vi "RTS Door Operation Routine.vi"(4 "Relay Number":u8=1 min=1 max=3 step=1, 6 "Station #":u8=1 min=1 max=8 step=1, 8 "Error In":errorcluster, 11 "Door Opening Controller Input":T1 {"Chamber 1-1"."Start Time" format="%<%X\n%x>T"; "Chamber 1-1"."End Time" format="%<%X\n%x>T"; "Time Count (s)" format="%.2f"}) -> (0 "Error Out":errorcluster, 3 "Door Opening Controller Output":T1 {"Chamber 1-1"."Start Time" format="%<%X\n%x>T"; "Chamber 1-1"."End Time" format="%<%X\n%x>T"; "Time Count (s)" format="%.2f"})   [LabVIEW 2016]
uses:
  Type Definitions/RTS Door Opener Indicator.ctl
  Type Definitions/RTS Door Ops Client.ctl
  Type Definitions/RTS Door Opening Schedule.ctl
  Type Definitions/RTS Door Ops Sequence.ctl
panel:
  # "Chamber Conditions:"
  # "Chamber Conditions:"
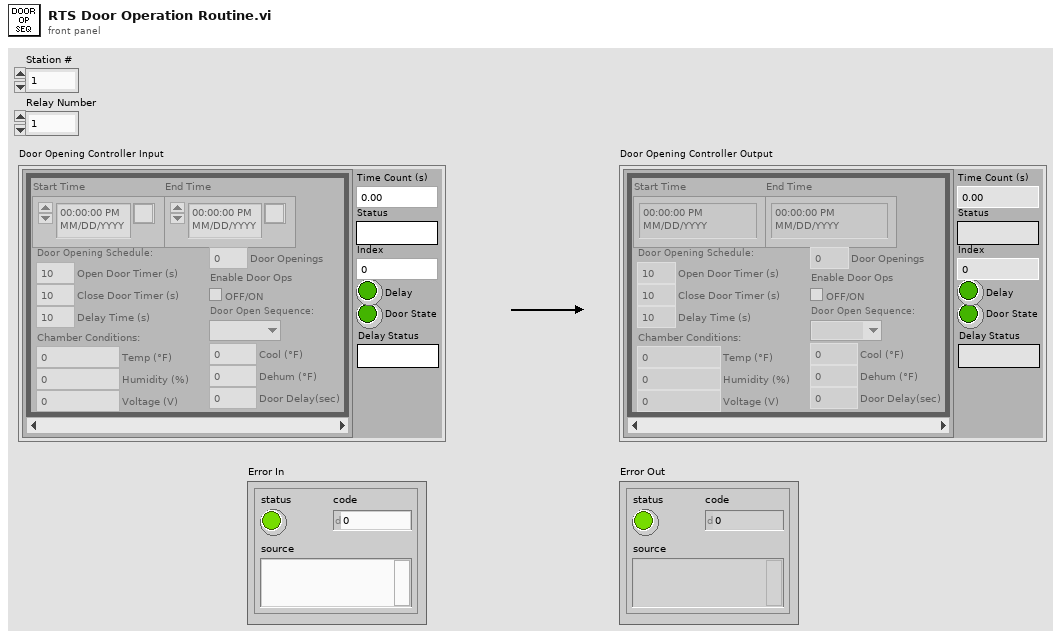
[diagram p1: front panel]
types:
  T1 = typedef "RTS Door Opener Indicator.ctl" = cluster{"Time Count (s)":dbl, "Status":string, "Door State":bool, "Delay":bool, "Chamber 1-1":T2[], "Index":i32, "Delay Status":string}
  T2 = typedef "RTS Door Ops Client.ctl" = cluster{"End Time":timestamp, "Start Time":timestamp, "Door Opening Schedule:":T3, "Enable Door Ops":bool, "Door Openings":u32, "Temp (°F)":dbl, "Humidity (%)":dbl, "Voltage (V)":dbl, "Door Open Sequence:":T4, "Door Delay(sec)":dbl, "Dehum (°F)":dbl, "Cool (°F)":dbl}
  T3 = typedef "RTS Door Opening Schedule.ctl" = cluster{"Open Door Timer (s)":dbl, "Delay Time (s)":dbl, "Close Door Timer (s)":dbl}
  T4 = typedef "RTS Door Ops Sequence.ctl" = enum16{"", "1st", "2nd", "3rd"}
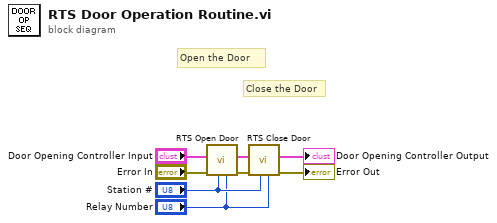
[diagram p0: block diagram]
diagram:
  # "Close the Door"
  # "Open the Door"
  n1 = call "RTS Open Door.vi"("Relay Number"="Relay Number", "Station #"="Station #", "Error In"="Error In", "Door Opening Controller Input"="Door Opening Controller Input") -> ("Error Out"=w7:errorcluster, "Door Opening Controller Output"=w6:T1)  [unwired: 6 in]
  n2 = call "RTS Close Door.vi"("Relay Number"="Relay Number", "Station #"="Station #", "Error In"=w7, "Door Opening Controller Input"=w6) -> ("Error Out"=→"Error Out":errorcluster, "Door Opening Controller Output"=→"Door Opening Controller Output":T1)  [unwired: 6 in]
